vi "process switch state.vi"(7 "Close?":bool, 8 "error in (no error)":errorcluster, 10 "List":refnum<class "Relay.lvclass">[](array[class]), 11 "Session Handle in":T1) -> (0 "error out":errorcluster, 3 "Session Handle out":T1)   [LabVIEW 2015, in "SLSC Switch.lvlib" / "Switch Action Processor.lvclass"]
uses:
  Switch Action Processor.lvclass
  Relay/Relay.lvclass
  SLSC Session/Typedefs/Session Handle.ctl
  SLSC Session/SLSC Session.lvclass
  <vilib>/SLSC/Flatten Names (String).vi
  <vilib>/SLSC/SLSC.lvlib
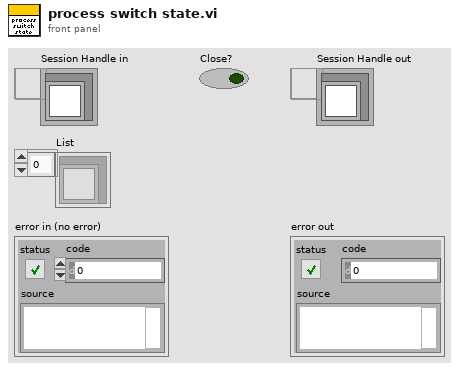
[diagram p1: front panel]
types:
  T1 = typedef "SLSC Switch.lvlib/SLSC Session.lvclass/Session Handle.ctl" = refnum<data-value>
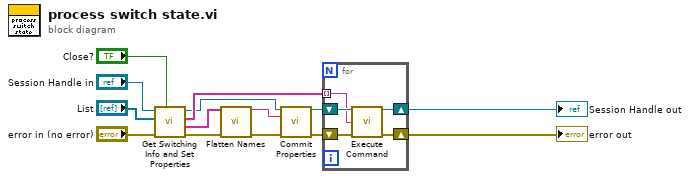
[diagram p0: block diagram]
diagram:
  n1 = call "Get Switching Info and Set Properties.vi"("Close?"="Close?", "error in (no error)"="error in (no error)", "Relays"="List", "SLSC Session In"="Session Handle in") -> ("error out"=w10:errorcluster, "property resources"=w4:string[], "commands"=w7:string[], "SLSC Session Out"=w2:T1)  [unwired: 4 in]
  n2 = call-poly <vilib>:"Flatten Names.vi"("names in"=w4, "error in (no error)"=w10) -> ("names out"=w3:string, "error out"=w9:errorcluster)  [unwired: 12 in]
  n3 = call "Commit Properties.vi"("Session Handle in"=w2, "resources"=w3, "error in (no error)"=w9) -> ("Session Handle out"=w6:T1, "error out"=w12:errorcluster)  [unwired: 11 in]
  n4 = for {
    tunnel: w7 -> [w18] mode=indexing
    shift-right: [w16] -> w13
    shift-left: w12 -> [w17]
    shift-right: [w15] -> w1
    shift-left: w6 -> [w19]
    n5 = call "Execute Command.vi"("Session Handle in"=w19, "command"=w18, "error in (no error)"=w17) -> ("Session Handle out"=w15:T1, "error out"=w16:errorcluster)  [unwired: 11 in]
  }
  "error out" <- w13
  "Session Handle out" <- w1
